vi "New.vi"(8 "Error In":errorcluster) -> (0 "Error Out":errorcluster, 3 "Renderer":refnum<class "Renderer.lvclass">)   [LabVIEW 2018, in "Toolkit.lvlib" / "Renderer.lvclass"]
uses:
  Renderer.lvclass
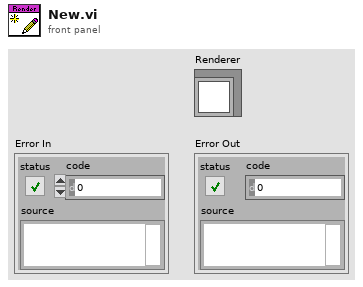
[diagram p1: front panel]
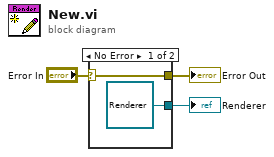
[diagram p0: block diagram]
diagram:
  n1 = case shown="No Error" "Error In" {
    selector: "Error In" -> [w5 w6]
    tunnel: [w5 w6] -> w2
    tunnel: [refnum<class "Renderer.lvclass"> refnum ("Toolkit.lvlib:Renderer.lvclass") _] -> w1
    frame No Error {
    }
    frame Error {
    }
  }
  "Error Out" <- w2
  "Renderer" <- w1
